vi "CRYGetWaterMark.vi"(8 "Type":string, 9 "Offset_Y":i16, 10 "Offset_X":i16, 11 "Plot Area Bounds":T1) -> (3 "WaterMark Image":picture)   [LabVIEW 2013]
uses:
  <vilib>/Utility/miscctls.llb/LVRectTypeDef.ctl
  CRYCurveLibrary/Global/CRYCurve Library Global.vi
  CRYMainGlobal.vi
panel:
  out "Image Index":i16
  in  "text color":u32(colorbox)=1149184
  in  "text orientation":T2(ring)
  in  "WaterMarkText":string="GV-Tech"
  in  "[user-specified font]":T3={"Font Name:"="Bradley Hand ITC", "Size"=26, "Strikeout?"=FALSE, "Italic?"=TRUE, "Underline?"=FALSE, "Outline?"=TRUE, "Shadow?"=TRUE, "Bold?"=TRUE}
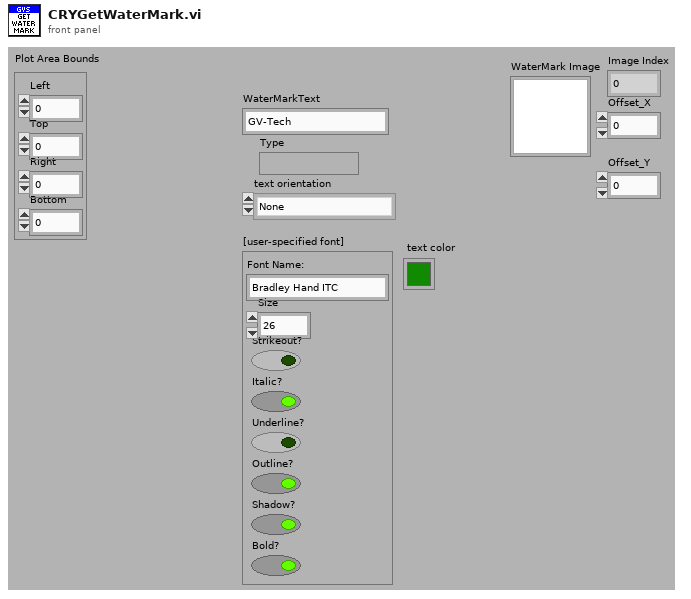
[diagram p1: front panel]
types:
  T1 = typedef "LVRectTypeDef.ctl" = cluster{"Left":i16, "Top":i16, "Right":i16, "Bottom":i16}
  T2 = enum16{"None", "Stacked", "Clockwise", "Counterclockwise"}
  T3 = cluster{"Font Name:":string, "Size":i16, "Strikeout?":bool, "Italic?":bool, "Underline?":bool, "Outline?":bool, "Shadow?":bool, "Bold?":bool}
  T4 = cluster{"horizontal":enum16{"left", "center", "right"}, "vertical":enum16{"top", "center", "bottom"}}
  T5 = enum16{"User-specified Font", "Application Font", "System Font", "Dialog Font"}
  T6 = enum32{"English", "Chinese", "Korean", "Japanese", "Russian", "Chinese traditional"}
  T7 = typedef "CRYImageData.ctl" = cluster{"image type":i32, "image depth":i32, "image":u8[], "mask":u8[], "colors":u32[], "Rectangle":cluster{"left":i16, "top":i16, "right":i16, "bottom":i16}}
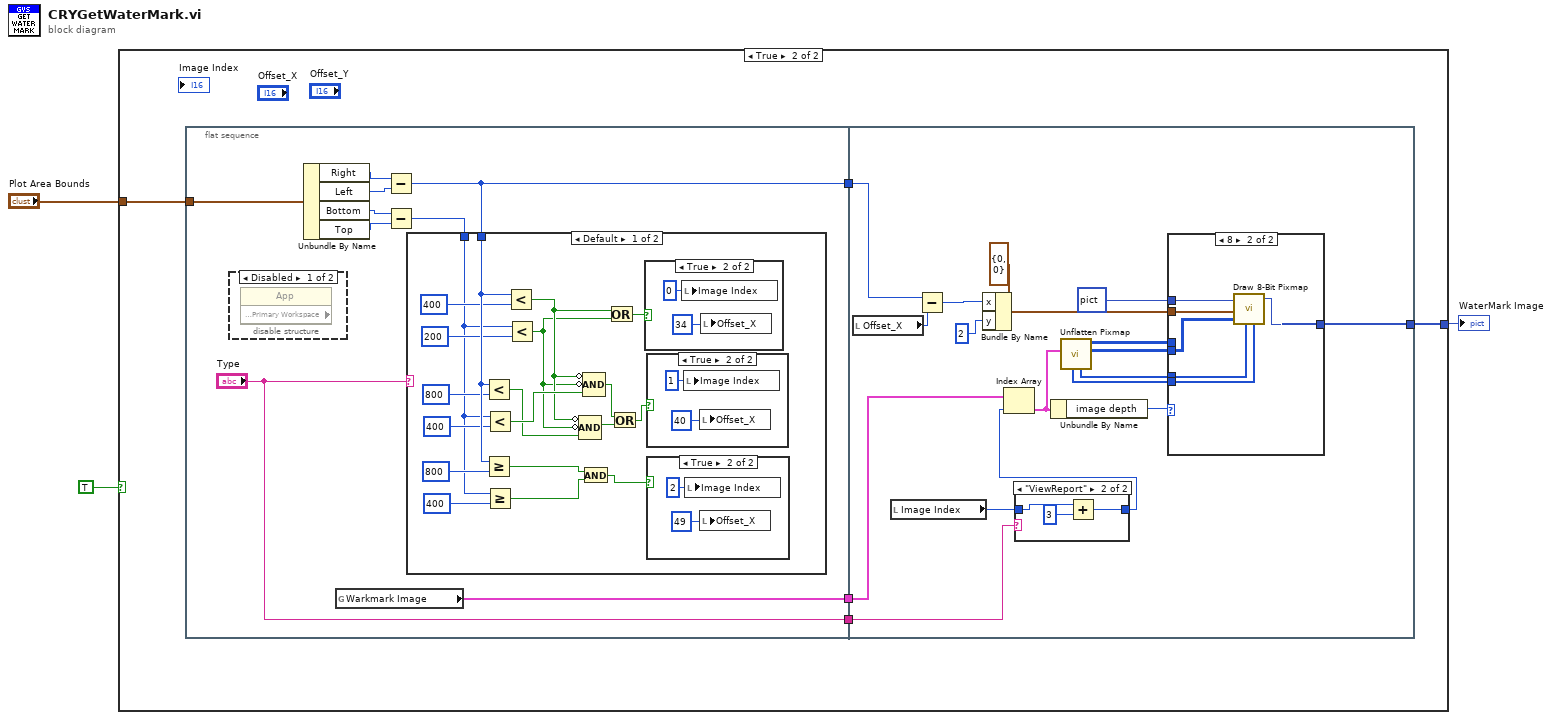
[diagram p0: block diagram]
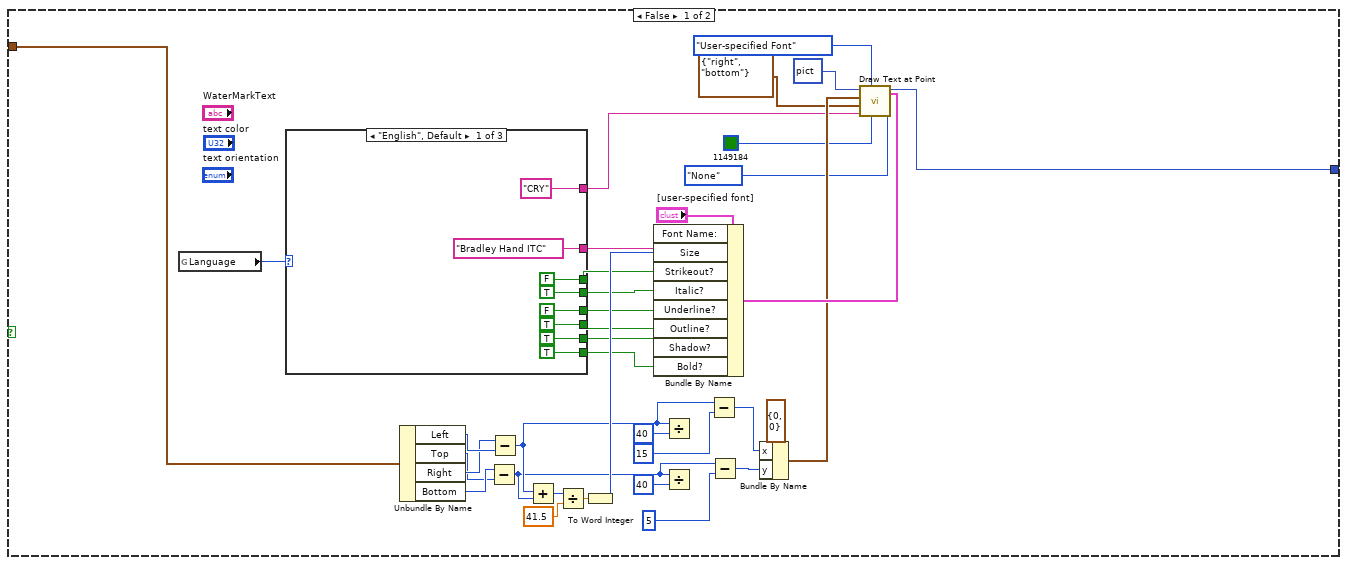
[diagram p2: hidden frame]
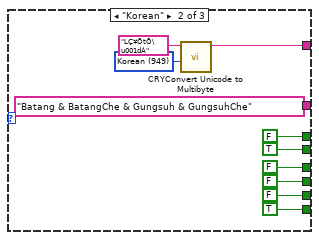
[diagram p3: hidden frame]
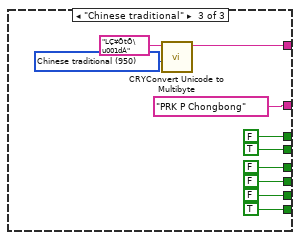
[diagram p4: hidden frame]
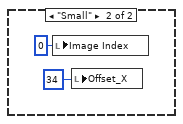
[diagram p8: hidden frame]
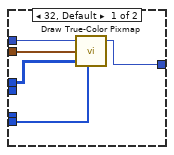
[diagram p11: hidden frame]
diagram:
  n1 = case shown="True" TRUE {
    tunnel: [w27 w69] -> w3
    tunnel: "Plot Area Bounds" -> [w4 w72]
    frame False {
      n2 = global read "CRYMainGlobal.vi" "Language"() -> (w13:T6)
      n3 = case shown="\"English\", Default" w13 {
        tunnel: ["Bradley Hand ITC" ("Font Name:") "Batang & BatangChe & Gungsuh & GungsuhChe" ("Font Name:") "PRK P Chongbong" ("Font Name:")] -> w12
        tunnel: ["CRY" ("WaterMarkText") w50 w60] -> w11
        tunnel: [FALSE ("Strikeout?") FALSE ("Strikeout?") FALSE ("Strikeout?")] -> w10
        tunnel: [TRUE ("Italic?") TRUE ("Italic?") TRUE ("Italic?")] -> w9
        tunnel: [FALSE ("Underline?") FALSE ("Underline?") FALSE ("Underline?")] -> w8
        tunnel: [TRUE ("Outline?") FALSE ("Outline?") FALSE ("Outline?")] -> w7
        tunnel: [TRUE ("Shadow?") FALSE ("Shadow?") FALSE ("Shadow?")] -> w6
        tunnel: [TRUE ("Bold?") TRUE ("Bold?") TRUE ("Bold?")] -> w5
        frame "English", Default {
        }
        frame "Korean" {
          w48 = 949 items=["System default"=0, "Latin-1"=1252, "Japanese"=932, "Korean"=949, "Chinese simplified"=936, "Chinese traditional"=950, "Central Europe"=1250, "Cyrillic"=1251, "Greek"=1253, "Turkish"=1254, "Hebrew"=1255, "Arabic"=1256, "Baltic"=1257, "Thai"=874, "Vietnamese"=783, "UTF8"=65001, "UTF-7"=65000] ("Code Page")
          n4 = call "CRYConvert Unicode to Multibyte.vi"("Code Page"=w48, "Unicode String"="LÇ¥ÕtÕ\u001dÁ") -> ("Multibyte string"=w50:string)  [unwired: 8 in, 1 out]
        }
        frame "Chinese traditional" {
          w58 = 950 items=["System default"=0, "Latin-1"=1252, "Japanese"=932, "Korean"=949, "Chinese simplified"=936, "Chinese traditional"=950, "Central Europe"=1250, "Cyrillic"=1251, "Greek"=1253, "Turkish"=1254, "Hebrew"=1255, "Arabic"=1256, "Baltic"=1257, "Thai"=874, "Vietnamese"=783, "UTF8"=65001, "UTF-7"=65000] ("Code Page")
          n5 = call "CRYConvert Unicode to Multibyte.vi"("Code Page"=w58, "Unicode String"="LÇ¥ÕtÕ\u001dÁ") -> ("Multibyte string"=w60:string)  [unwired: 8 in, 1 out]
        }
      }
      n6 = Unbundle By Name(w4) -> ("Left"=w38:i16, "Top"=w35:i16, "Right"=w36:i16, "Bottom"=w37:i16)
      n7 = Subtract(x=w37, y=w35) -> (x-y=w20:i16)
      n8 = Subtract(x=w36, y=w38) -> (x-y=w22:i16)
      n9 = Add(x=w22, y=w20) -> (x+y=w32:i16)
      n10 = Divide(x=w32, y=41.5) -> (x/y=w31:dbl)
      n11 = To Word Integer(number=w31) -> (16bit integer=w30:i16)
      n12 = Bundle By Name(cluster="[user-specified font]", "Font Name:"=w12, "Size"=w30, "Strikeout?"=w10, "Italic?"=w9, "Underline?"=w8, "Outline?"=w7, "Shadow?"=w6, "Bold?"=w5) -> (w29:T3)
      n13 = Divide(x=w22, y=i16 40) -> ()  [unwired: 1 out]
      n14 = Divide(x=w20, y=i16 40) -> ()  [unwired: 1 out]
      n15 = Subtract(x=w22, y=i16 15) -> (x-y=w21:i16)
      n16 = Subtract(x=w20, y=i16 5) -> (x-y=w19:i16)
      n17 = Bundle By Name(cluster=cluster{"x":i16, "y":i16} {"x"=0, "y"=0} ("origin"), "x"=w21, "y"=w19) -> (w25:cluster{"x":i16, "y":i16})
      n18 = call <vilib>:"Draw Text at Point.vi"("text orientation"=T2."None", "[user-specified font]"=w29, "text color(black)"=u32 1149184 ("text color"), "desired font(Application)"=T5."User-specified Font", "text"=w11, "alignment(left, top)"=T4 {"horizontal"=enum."right", "vertical"=enum."bottom"}, "origin"=w25, "picture"=picture data[5B] ("Plot Images:Front")) -> ("new picture"=w27:picture)  [unwired: 1 in, 2 out]
    }
    frame True {
      n19 = flat-sequence {
        tunnel: w72 -> [w81]
        tunnel: [w79] -> w71
        tunnel: [w80] -> w70
        tunnel: ["Type"] -> w68
        tunnel: w71 -> [w124]
        tunnel: w70 -> [w123]
        tunnel: [w121] -> w69
        tunnel: w68 -> [w111]
        frame #0 {
          n20 = disable-structure shown="Disabled" {
            frame Disabled {
              n21 = property class="App" props=["Display:Primary Workspace"]() -> ()  [unwired: 2 in, 3 out]
            }
            frame Enabled {
            }
          }
          n22 = Unbundle By Name(w81) -> ("Right"=w78:i16, "Left"=w77:i16, "Bottom"=w76:i16, "Top"=w75:i16)
          n23 = global read "CRYCurve Library Global.vi" "Warkmark Image"() -> (w79:T7[])
          n24 = Subtract(x=w78, y=w77) -> (x-y=w80:i16)
          n25 = Subtract(x=w76, y=w75) -> (x-y=w74:i16)
          n26 = case shown="Default" "Type" {
            tunnel: w80 -> [w100 _]
            tunnel: w74 -> [w92 _]
            frame Default {
              n27 = Less?(x=w100, y=i16 800) -> (x < y?=w86:bool)
              n28 = Greater Or Equal?(x=w100, y=i16 800) -> (x >= y?=w90:bool)
              n29 = Less?(x=w92, y=i16 400) -> (x < y?=w91:bool)
              n30 = Greater Or Equal?(x=w92, y=i16 400) -> (x >= y?=w89:bool)
              n31 = Less?(x=w100, y=i16 400) -> (x < y?=w87:bool)
              n32 = Less?(x=w92, y=i16 200) -> (x < y?=w85:bool)
              n33 = Compound Arithmetic op=AND(invert w87, invert w85, w86) -> (w83:bool)
              n34 = And(x=w90, y=w89) -> (x .and. y?=w88:bool)
              n35 = Compound Arithmetic op=AND(invert w87, invert w85, w91) -> (w84:bool)
              n36 = Or(x=w87, y=w85) -> (x .or. y?=w97:bool)
              n37 = Or(x=w84, y=w83) -> (x .or. y?=w82:bool)
              n38 = case shown="True" w97 {
                frame False {
                }
                frame True {
                  n39 = local write "Image Index"(i16 0 ("Image Index")) -> ()
                  n40 = local write "Offset_X"(i16 34 ("y")) -> ()
                }
              }
              n41 = case shown="True" w82 {
                frame False {
                }
                frame True {
                  n42 = local write "Image Index"(i16 1 ("Image Index")) -> ()
                  n43 = local write "Offset_X"(i16 40 ("y")) -> ()
                }
              }
              n44 = case shown="True" w88 {
                frame False {
                }
                frame True {
                  n45 = local write "Image Index"(i16 2 ("Image Index")) -> ()
                  n46 = local write "Offset_X"(i16 49 ("y")) -> ()
                }
              }
            }
            frame "Small" {
              n47 = local write "Image Index"(i16 0 ("Image Index")) -> ()
              n48 = local write "Offset_X"(i16 34 ("y")) -> ()
            }
          }
        }
        frame #1 {
          n49 = local read "Offset_X"() -> (w122:i16)
          n50 = local read "Image Index"() -> (w110:i16)
          n51 = Subtract(x=w123, y=w122) -> (x-y=w125:i16)
          n52 = Bundle By Name(cluster=cluster{"x":i16, "y":i16} {"x"=0, "y"=0} ("origin"), "x"=w125, "y"=i16 2) -> (w126:cluster{"x":i16, "y":i16})
          n53 = case shown="\"ViewReport\"" w111 {
            tunnel: w110 -> [w127 w129]
            tunnel: [w127 w130] -> w109
            frame Default {
            }
            frame "ViewReport" {
              n54 = Add(x=w129, y=i16 3) -> (x+y=w130:i16)
            }
          }
          n55 = Index Array(array=w124, index=w109) -> (element=w116:T7)
          n56 = Unbundle By Name(w116) -> ("image depth"=w115:i32)
          n57 = call <vilib>:"Unflatten Pixmap.vi"("image data"=w116) -> ("8-bit pixmap"=w112:u8[][], "24-bit pixmap"=w117:u32[][], "colors"=w119:u32[], "mask"=w118:u8[])  [unwired: 4 in, 3 out]
          n58 = case shown="8" w115 {
            tunnel: w126 -> [w135 w141]
            tunnel: [w134 w140] -> w121
            tunnel: picture data[5B] ("picture") -> [w133 w139]
            tunnel: w119 -> [_ w138]
            tunnel: w118 -> [w132 w137]
            tunnel: w117 -> [w131 _]
            tunnel: w112 -> [_ w136]
            frame 32, Default {
              n59 = call <vilib>:"Draw True-Color Pixmap.vi"("picture"=w133, "top left point(0, 0)"=w135, "data (RGB format)"=w131, "mask"=w132) -> ("new picture"=w134:picture)  [unwired: 5 in]
            }
            frame 8 {
              n60 = call <vilib>:"Draw 8-Bit Pixmap.vi"("picture"=w139, "top left point(0, 0)"=w141, "data"=w136, "color table"=w138, "mask"=w137) -> ("new picture"=w140:picture)  [unwired: 4 in]
            }
          }
        }
      }
    }
  }
  "WaterMark Image" <- w3
